vi "SubVI Tester.vi"() -> ()   [LabVIEW 2012]
doc: "在高难练习中，将添加风信息至气象数据自定义类型。"
uses:
  Weather Data.ctl
panel:
  out "气象数据输出":T1={"当前温度"=0.0, "最高温度"=0.0, "最低温度"=0.0, "温度警告？"=FALSE, "温度警告文本"="无警告", "当前风速"=0.0, "最大风速"=0.0, "风速警告？"=FALSE, "风速警告文本"="无警告"}
  in  "最大风速":dbl
  in  "当前风速":dbl
  in  "最低温度":dbl
  in  "最高温度":dbl
  in  "停止":bool
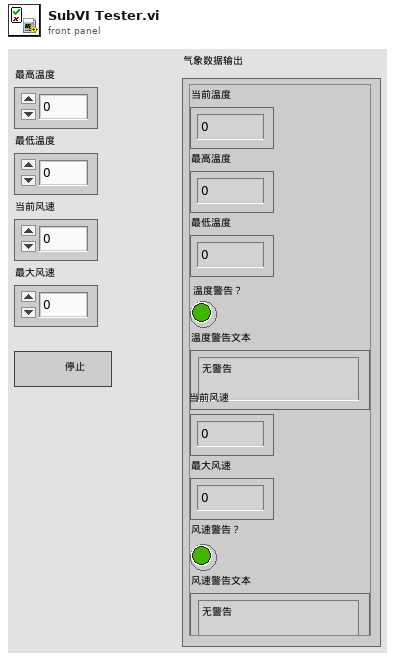
[diagram p1: front panel]
types:
  T1 = typedef "Weather Data.ctl" = cluster{"当前温度":dbl, "最高温度":dbl, "最低温度":dbl, "温度警告？":bool, "温度警告文本":string, "当前风速":dbl, "最大风速":dbl, "风速警告？":bool, "风速警告文本":string}
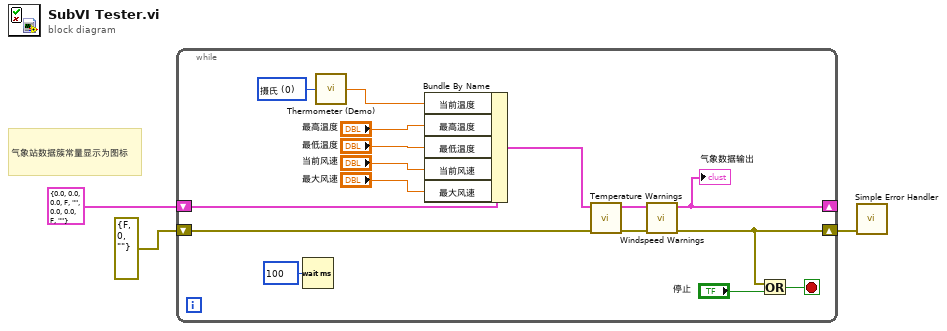
[diagram p0: block diagram]
diagram:
  # "气象站数据簇常量显示为图标"
  n1 = while {
    shift-right: [w12] -> _
    shift-left: T1 {"当前温度"=0.0, "最高温度"=0.0, "最低温度"=0.0, "温度警告？"=FALSE, "温度警告文本"="", "当前风速"=0.0, "最大风速"=0.0, "风速警告？"=FALSE, "风速警告文本"=""} ("气象数据输入") -> [w19]
    shift-right: [w13] -> w2
    shift-left: cluster{"状态":bool, "代码":i32, "源":string} {"状态"=FALSE, "代码"=0, "源"=""} ("错误输出") -> [w15]
    stop <- w16 stop-if-true
    w4 = u16 0 items=["摄氏", "华氏"] ("单位（0：摄氏度）")
    n2 = Wait (ms) ("等待(ms)")(milliseconds to wait=u32 100 ("等待时间（毫秒）")) -> ()  [unwired: 1 out]
    n3 = call "Thermometer (Demo).vi"("单位（0：摄氏度）"=w4) -> ("温度值"=w5:dbl)
    n4 = Bundle By Name ("按名称捆绑")(cluster=w19, "当前温度"=w5, "最高温度"="最高温度", "最低温度"="最低温度", "当前风速"="当前风速", "最大风速"="最大风速") -> (w11:T1)
    n5 = call "Temperature Warnings.vi"("错误输入"=w15, "气象数据输入"=w11) -> ("错误输出"=w14:cluster{"状态":bool, "代码":i32, "源":string}, "气象数据输出"=w10:T1)  [unwired: 8 in]
    n6 = call "Windspeed Warnings.vi"("错误输入"=w14, "气象数据输入"=w10) -> ("错误输出"=w13:cluster{"状态":bool, "代码":i32, "源":string}, "气象数据输出"=w12:T1)  [unwired: 8 in]
    "气象数据输出" <- w12
    n7 = Or ("或")(x=w13, y="停止") -> (x .or. y?=w16:bool)
  }
  n8 = call <vilib>:"Simple Error Handler.vi"("error in (no error)"=w2) -> ()  [unwired: 4 in, 5 out]
